vi "State_Send_Flows.vi"(7 "Mode":enum16{"User flows", "Auto flows"}(ring), 8 "User flows in":dbl[](array[numeric]), 9 "Auto flows in":dbl[][](array[numeric])) -> (3 "BBB command out":string)   [LabVIEW 2025]
uses:
  BBB/TypeDef_BBBJSON_commands.ctl
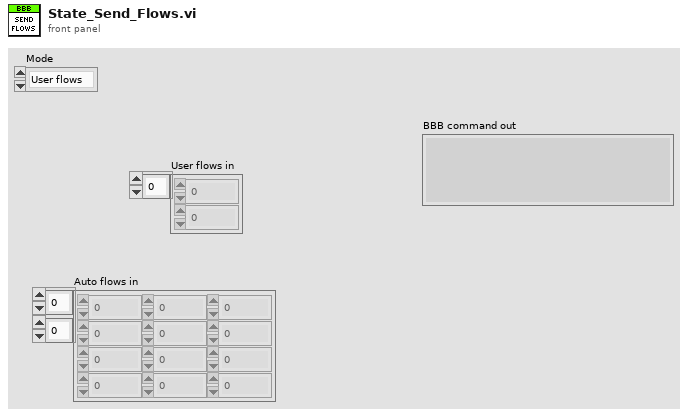
[diagram p1: front panel]
types:
  T1 = typedef "TypeDef_BBBJSON_commands.ctl" = cluster{"SetState":cluster{"StateNum":i32}, "SetSave":cluster{"Save":i16}, "SetTEC":cluster{"TargetT":dbl, "Reset":i32, "Enable":i32}, "SetMFC":cluster{"MFC0":dbl, "MFC1":dbl}, "SetGPIO":cluster{"SSR0":i16, "SSR1":i16, "LED":i16}}
  T2 = cluster{"SetMFC":cluster{"MFC0":dbl, "MFC1":dbl}}
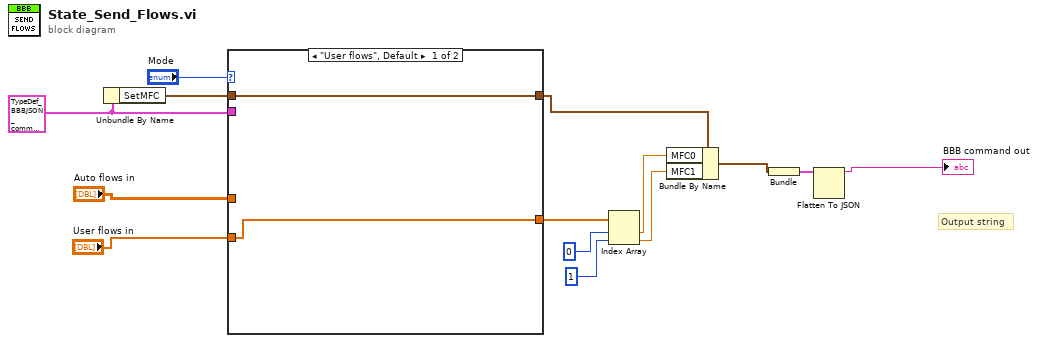
[diagram p0: block diagram]
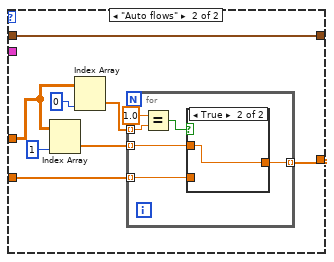
[diagram p2: hidden frame]
diagram:
  w2 = T1 {"SetState"={"StateNum"=0}, "SetSave"={"Save"=0}, "SetTEC"={"TargetT"=0.0, "Reset"=0, "Enable"=0}, "SetMFC"={"MFC0"=0.0, "MFC1"=0.0}, "SetGPIO"={"SSR0"=0, "SSR1"=0, "LED"=0}} ("BBBcommands")
  # "Output string"
  n1 = Unbundle By Name(w2) -> ("SetMFC"=w6:cluster{"MFC0":dbl, "MFC1":dbl})
  n2 = case shown="\"User flows\", Default" "Mode" {
    tunnel: "Auto flows in" -> [_ w22]
    tunnel: "User flows in" -> [w15 w19]
    tunnel: w2 -> [_ _]
    tunnel: [w15 w18] -> w11
    tunnel: w6 -> [w16 w17]
    tunnel: [w16 w17] -> w5
    frame "User flows", Default {
    }
    frame "Auto flows" {
      n3 = Index Array(array=w22, index (col)=1 ("disabled index (col)")) -> (element=w20:dbl[])  [unwired: 1 in]
      n4 = Index Array(array=w22, index (col)=0 ("disabled index (col)")) -> (element=w21:dbl[])  [unwired: 1 in]
      n5 = for {
        tunnel: w21 -> [w27] mode=indexing
        tunnel: w20 -> [w30] mode=indexing
        tunnel: w19 -> [w29] mode=indexing
        tunnel: [w28] -> w18 mode=indexing
        n6 = Equal?(x=1.0, y=w27) -> (x = y?=w25:bool)
        n7 = case shown="True" w25 {
          tunnel: w30 -> [_ w32]
          tunnel: w29 -> [w31 _]
          tunnel: [w31 w32] -> w28
          frame False {
          }
          frame True {
          }
        }
      }
    }
  }
  n8 = Index Array(array=w11, index #1=0 ("index"), index #2=1 ("index")) -> (element #1=w8:dbl, element #2=w7:dbl)
  n9 = Bundle By Name(cluster=w5, "MFC0"=w8, "MFC1"=w7) -> (w12:cluster{"MFC0":dbl, "MFC1":dbl})
  n10 = Bundle("SetMFC"=w12) -> (w13:T2)  [unwired: 1 in]
  n11 = Flatten To JSON(anything=w13) -> (JSON string=→"BBB command out":string)  [unwired: 2 in, 1 out]
